vi "To Package Name.vi"(0 "Package Name":string, 11 "error in (no error)":errorcluster) -> (4 "Valid Package Name":string, 15 "error out":errorcluster)   [LabVIEW 2021, in "Measurement Builder.lvlib"]
uses:
  Measurement Builder.lvlib
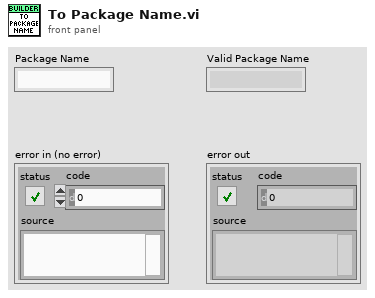
[diagram p1: front panel]
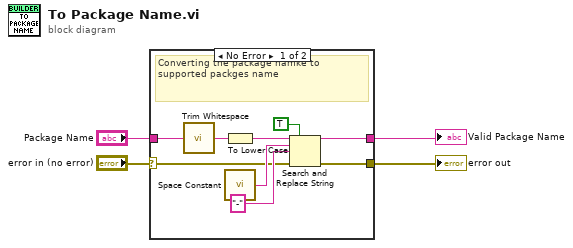
[diagram p0: block diagram]
diagram:
  n1 = case shown="No Error" "error in (no error)" {
    selector: "error in (no error)" -> [w7 w14]
    tunnel: [w12 w14] -> w4
    tunnel: [w11 _] -> w3
    tunnel: "Package Name" -> [w6 _]
    frame No Error {
      # "Converting the package namke to supported packges name"
      n2 = call <vilib>:"Trim Whitespace.vi"("string"=w6) -> ("trimmed string"=w5:string)  [unwired: 1 in]
      n3 = To Lower Case(string=w5) -> (all lower case string=w8:string)
      n4 = call <vilib>:"Space Constant.vi"() -> ("String"=w9:string)
      n5 = Search and Replace String(replace all?=TRUE ("replace all? (F)"), input string=w8, search string=w9, replace string="-" ("replace string (\"\")"), error in=w7) -> (result string=w11:string, error out=w12:errorcluster)  [unwired: 3 in, 2 out]
    }
    frame Error {
    }
  }
  "error out" <- w4
  "Valid Package Name" <- w3
